vi "Take_it.vi"(8 "error in (no error) 2":errorcluster, 10 "Combo Box":string(combo), 11 "Camera Image":T1) -> (0 "error out":errorcluster, 2 "Done":bool)   [LabVIEW 2019]
uses:
  <vilib>/vision/Image Controls.llb/IMAQ Image.ctl
  Mashina_podyehala.vi
  Camera_angle.vi
  Arm_stage_var.vi
  Timer.vi
  <vilib>/vision/NI_Vision_Development_Module.lvlib
  Simulated Robot/Simulation SubVIs/Simulation SubVIs.lvlib
panel:
  out "New Image":T1
  out "Stage":i32
  out "Threshold":T1(plugin-control)
  out "Raw Image":T1(plugin-control)
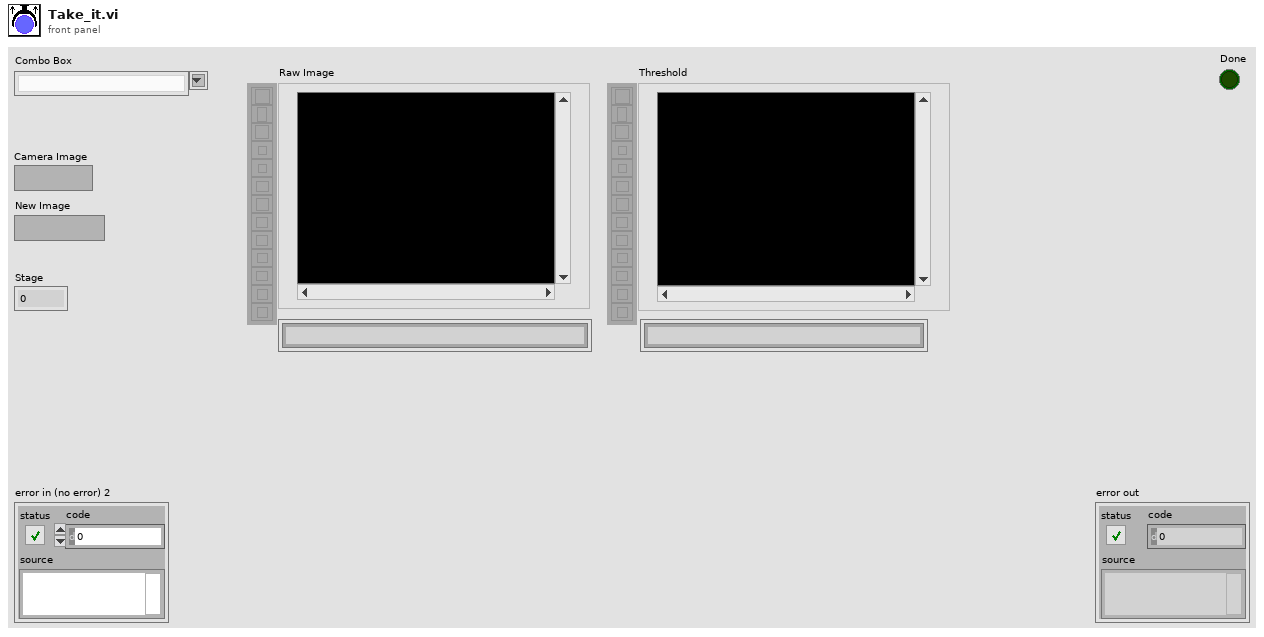
[diagram p1: front panel]
types:
  T1 = typedef "IMAQ Image.ctl" = refnum<image>
  T2 = typedef "Image Type" = u32
  T3 = typedef "Particle Parameters" = i32
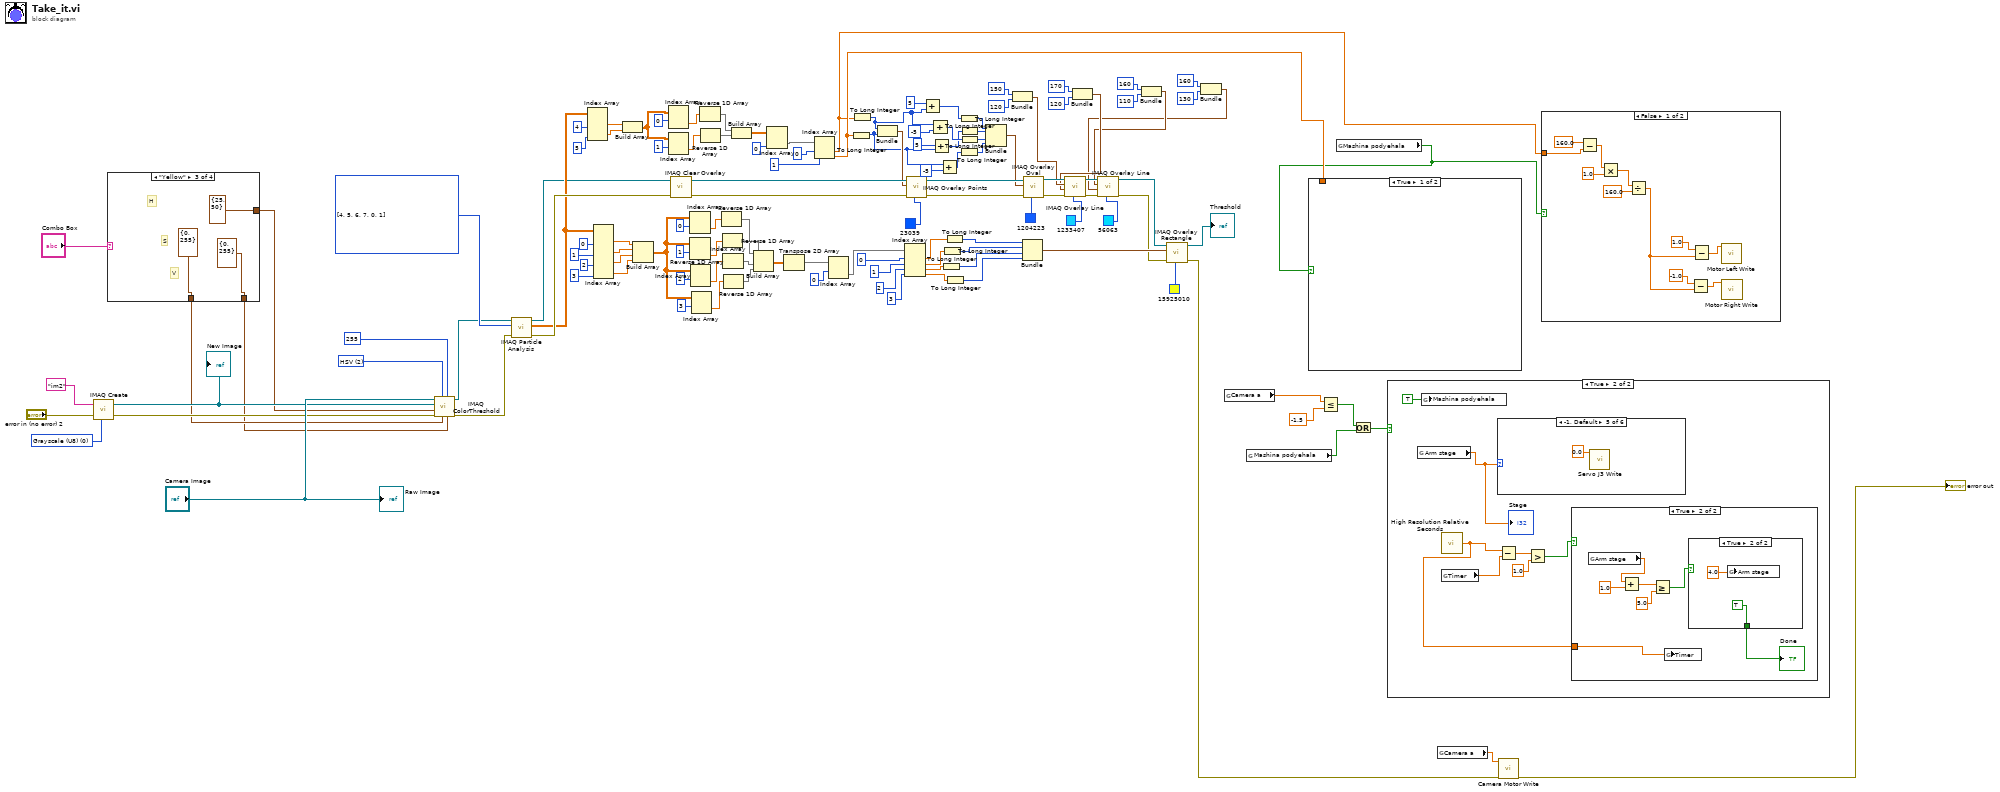
[diagram p0: block diagram]
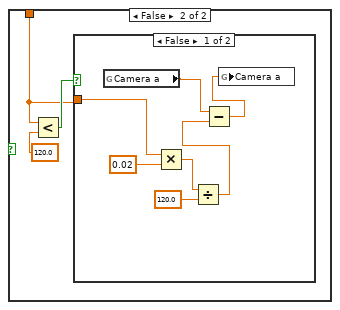
[diagram p2: hidden frame]
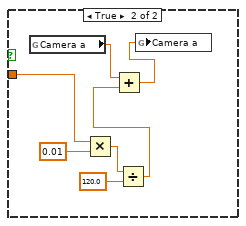
[diagram p3: hidden frame]
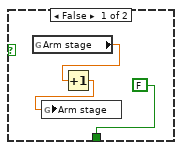
[diagram p6: hidden frame]
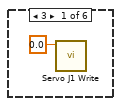
[diagram p7: hidden frame]
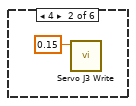
[diagram p8: hidden frame]
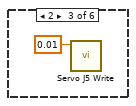
[diagram p9: hidden frame]
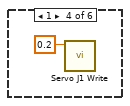
[diagram p10: hidden frame]
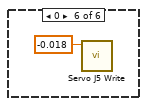
[diagram p11: hidden frame]
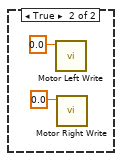
[diagram p12: hidden frame]
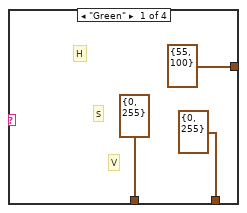
[diagram p13: hidden frame]
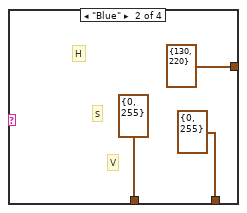
[diagram p14: hidden frame]
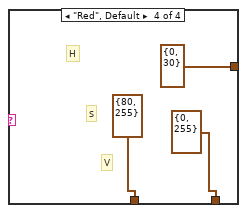
[diagram p15: hidden frame]
diagram:
  w13 = T2 0 items=["Grayscale (U8)", "Grayscale (I16)", "Grayscale (SGL)", "Complex (CSG)", "RGB (U32)", "HSL (U32)", "RGB (U64)", "Grayscale (U16)"] ("Image Type")
  w126 = u16 2 items=["RGB", "HSL", "HSV", "HSI"] ("Color Mode")
  w124 = T3[] [4, 5, 6, 7, 0, 1] items=["Center of Mass X", "Center of Mass Y", "First Pixel X", "First Pixel Y", "Bounding Rect Left", "Bounding Rect Top", "Bounding Rect Right", "Bounding Rect Bottom", "Max Feret Diameter Start X", "Max Feret Diameter Start Y", "Max Feret Diameter End X", "Max Feret Diameter End Y", "Max Horiz. Segment Length Left", "Max Horiz. Segment Length Right", "Max Horiz. Segment Length Row", "-", "Bounding Rect Width", "Bounding Rect Height", "Bounding Rect Diagonal", "Perimeter", "Convex Hull Perimeter", "Holes' Perimeter", "Max Feret Diameter", "Equivalent Ellipse Major Axis", "Equivalent Ellipse Minor Axis", "Equivalent Ellipse Minor Axis (Feret)", "Equivalent Rect Long Side", "Equivalent Rect Short Side", "Equivalent Rect Diagonal", "Equivalent Rect Short Side (Feret)", "Average Horiz. Segment Length", "Average Vert. Segment Length", "Hydraulic Radius", "Waddel Disk Diameter", "-", "Area", "Holes' Area", "Particle & Holes' Area", "Convex Hull Area", "Image Area", "-", "Number of Holes", "Number of Horiz. Segments", "Number of Vert. Segments", "-", "Orientation", "Max Feret Diameter Orientation", "-", "% Area/Image Area", "% Area/(Particle & Holes' Area)", "Ratio of Equivalent Ellipse Axes", "Ratio of Equivalent Rect Sides", "-", "Elongation Factor", "Compactness Factor", "Heywood Circularity Factor", "Type Factor", "-", "Sum X", "Sum Y", "Sum XX", "Sum XY", "Sum YY", "Sum XXX", "Sum XXY", "Sum XYY", "Sum YYY", "-", "Moment of Inertia XX", "Moment of Inertia XY", "Moment of Inertia YY", "Moment of Inertia XXX", "Moment of Inertia XXY", "Moment of Inertia XYY", "Moment of Inertia YYY", "Norm. Moment of Inertia XX", "Norm. Moment of Inertia XY", "Norm. Moment of Inertia YY", "Norm. Moment of Inertia XXX", "Norm. Moment of Inertia XXY", "Norm. Moment of Inertia XYY", "Norm. Moment of Inertia YYY", "Hu Moment 1", "Hu Moment 2", "Hu Moment 3", "Hu Moment 4", "Hu Moment 5", "Hu Moment 6", "Hu Moment 7"] ("Pixel Measurements")
  n1 = call "IMAQ Create"("Image Name"="im2", "Image Type"=w13, "error in (no error)"="error in (no error) 2") -> ("New Image"=w12:T1, "error out"=w9:errorcluster)  [unwired: 2 in]
  "New Image" <- w12
  n2 = case shown="\"Yellow\"" "Combo Box" {
    tunnel: [cluster{"Lower value":i32, "Upper value":i32} {"Lower value"=55, "Upper value"=100} ("Red or Hue Range") cluster{"Lower value":i32, "Upper value":i32} {"Lower value"=130, "Upper value"=220} ("Red or Hue Range") cluster{"Lower value":i32, "Upper value":i32} {"Lower value"=25, "Upper value"=50} ("Red or Hue Range") cluster{"Lower value":i32, "Upper value":i32} {"Lower value"=0, "Upper value"=30} ("Red or Hue Range")] -> w6
    tunnel: [cluster{"Lower value":i32, "Upper value":i32} {"Lower value"=0, "Upper value"=255} ("Green or Sat Range") cluster{"Lower value":i32, "Upper value":i32} {"Lower value"=0, "Upper value"=255} ("Green or Sat Range") cluster{"Lower value":i32, "Upper value":i32} {"Lower value"=0, "Upper value"=255} ("Green or Sat Range") cluster{"Lower value":i32, "Upper value":i32} {"Lower value"=80, "Upper value"=255} ("Green or Sat Range")] -> w5
    tunnel: [cluster{"Lower value":i32, "Upper value":i32} {"Lower value"=0, "Upper value"=255} ("Blue or Luma or Val or Inten Range") cluster{"Lower value":i32, "Upper value":i32} {"Lower value"=0, "Upper value"=255} ("Blue or Luma or Val or Inten Range") cluster{"Lower value":i32, "Upper value":i32} {"Lower value"=0, "Upper value"=255} ("Blue or Luma or Val or Inten Range") cluster{"Lower value":i32, "Upper value":i32} {"Lower value"=0, "Upper value"=255} ("Blue or Luma or Val or Inten Range")] -> w4
    frame "Green" {
      # "V"
      # "S"
      # "H"
    }
    frame "Blue" {
      # "V"
      # "S"
      # "H"
    }
    frame "Yellow" {
      # "V"
      # "S"
      # "H"
    }
    frame "Red", Default {
      # "V"
      # "S"
      # "H"
    }
  }
  n3 = call "IMAQ ColorThreshold"("Blue or Luma or Val or Inten Range"=w4, "Replace Value"=255, "Green or Sat Range"=w5, "Color Mode"=w126, "error in (no error)"=w9, "Red or Hue Range"=w6, "Image Dst"=w12, "Image Src"="Camera Image") -> ("error out"=w19:errorcluster, "Image Dst Out"=w8:T1)  [unwired: 2 in]
  n4 = call "IMAQ Particle Analysis"("error in (no error)"=w19, "Pixel Measurements"=w124, "Image"=w8) -> ("error out"=w25:errorcluster, "Particle Measurements (Pixels)"=w24:dbl[][], "Image Out (duplicate)"=w7:T1)  [unwired: 3 in, 3 out]
  n5 = Index Array(array=w24, index (col) #1=4 ("disabled index (col)"), index (col) #2=5 ("index (col)")) -> (element #1=w74:dbl[], element #2=w73:dbl[])  [unwired: 2 in]
  n6 = Index Array(array=w24, index (col) #1=0 ("disabled index (col)"), index (col) #2=1 ("index (col)"), index (col) #3=2 ("index (col)"), index (col) #4=3 ("index (col)")) -> (element #1=w119:dbl[], element #2=w118:dbl[], element #3=w117:dbl[], element #4=w116:dbl[])  [unwired: 4 in]
  n7 = Build Array(w74, w73) -> (w70:dbl[][])
  n8 = Build Array(w119, w118, w117, w116) -> (w107:dbl[][])
  n9 = Index Array(array=w70, index (row)=0) -> (element=w69:dbl[])  [unwired: 1 in]
  n10 = Index Array(array=w70, index (row)=1) -> (element=w68:dbl[])  [unwired: 1 in]
  n11 = call "IMAQ Clear Overlay"("error in (no error)"=w25, "Image"=w7) -> ("error out"=w63:errorcluster, "Image Out"=w80:T1)  [unwired: 8 in]
  n12 = Index Array(array=w107, index (row)=0) -> (element=w115:dbl[])  [unwired: 1 in]
  n13 = Index Array(array=w107, index (row)=1) -> (element=w114:dbl[])  [unwired: 1 in]
  n14 = Index Array(array=w107, index (row)=2) -> (element=w113:dbl[])  [unwired: 1 in]
  n15 = Index Array(array=w107, index (row)=3) -> (element=w108:dbl[])  [unwired: 1 in]
  n16 = Reverse 1D Array(array=w69) -> (reversed array=w67:dbl[])
  n17 = Reverse 1D Array(array=w68) -> (reversed array=w66:dbl[])
  n18 = Reverse 1D Array(array=w115) -> (reversed array=w111:dbl[])
  n19 = Reverse 1D Array(array=w114) -> (reversed array=w112:dbl[])
  n20 = Reverse 1D Array(array=w113) -> (reversed array=w110:dbl[])
  n21 = Reverse 1D Array(array=w108) -> (reversed array=w109:dbl[])
  n22 = Build Array(w67, w66) -> (w65:dbl[][])
  n23 = Build Array(w111, w112, w110, w109) -> (w102:dbl[][])
  n24 = Index Array(array=w65, index (col)=0 ("index (row)")) -> (element=w79:dbl[])  [unwired: 1 in]
  n25 = Transpose 2D Array(2D array=w102) -> (transposed array=w90:dbl[][])
  n26 = Index Array(array=w79, index #1=0 ("index"), index #2=1 ("index")) -> (element #1=w21:dbl, element #2=w22:dbl)
  n27 = Index Array(array=w90, index (row)=0) -> (element=w89:dbl[])  [unwired: 1 in]
  n28 = To Long Integer(number=w22) -> (32bit integer=w49:i32)
  n29 = To Long Integer(number=w21) -> (32bit integer=w52:i32)
  n30 = Bundle(w52, w49) -> (w75:cluster{i32, i32})  [unwired: 1 in]
  n31 = Index Array(array=w89, index #1=0 ("index"), index #2=1 ("index"), index #3=2 ("index"), index #4=3 ("index")) -> (element #1=w88:dbl, element #2=w87:dbl, element #3=w86:dbl, element #4=w85:dbl)
  n32 = call "IMAQ Overlay Points"("Color"=u32 23039, "error in (no error)"=w63, "Point"=w75, "Image"=w80) -> ("error out"=w62:errorcluster, "Image Out"=w64:T1)  [unwired: 6 in]
  n33 = Add(x=5, y=w52) -> (x+y=w54:i32)
  n34 = Add(x=w52, y=-5) -> (x+y=w53:i32)
  n35 = Add(x=5, y=w49) -> (x+y=w46:i32)
  n36 = Add(x=w49, y=-5) -> (x+y=w47:i32)
  n37 = To Long Integer(number=w86) -> (32bit integer=w93:i32)
  n38 = To Long Integer(number=w87) -> (32bit integer=w94:i32)
  n39 = To Long Integer(number=w88) -> (32bit integer=w95:i32)
  n40 = To Long Integer(number=w85) -> (32bit integer=w92:i32)
  n41 = To Long Integer(number=w54) -> (32bit integer=w56:i32)
  n42 = To Long Integer(number=w47) -> (32bit integer=w57:i32)
  n43 = To Long Integer(number=w46) -> (32bit integer=w59:i32)
  n44 = To Long Integer(number=w53) -> (32bit integer=w58:i32)
  n45 = Bundle(w56, w59, w58, w57) -> (w60:cluster{i32, i32, i32, i32})  [unwired: 1 in]
  n46 = Bundle(150, 120) -> (w35:cluster{i32, i32})  [unwired: 1 in]
  n47 = Bundle(w95, w94, w93, w92) -> (w96:cluster{i32, i32, i32, i32})  [unwired: 1 in]
  n48 = call "IMAQ Overlay Oval"("Color"=u32 1204223, "error in (no error)"=w62, "Bounding Rectangle"=w60, "Image"=w64) -> ("error out"=w44:errorcluster, "Image Out"=w45:T1)  [unwired: 6 in]
  n49 = Bundle(170, 120) -> (w32:cluster{i32, i32})  [unwired: 1 in]
  n50 = call "IMAQ Overlay Line"("Color"=u32 1233407, "error in (no error)"=w44, "End Point"=w32, "Start Point"=w35, "Image"=w45) -> ("error out"=w42:errorcluster, "Image Out"=w43:T1)  [unwired: 5 in]
  n51 = Bundle(160, 110) -> (w27:cluster{i32, i32})  [unwired: 1 in]
  n52 = Bundle(160, 130) -> (w26:cluster{i32, i32})  [unwired: 1 in]
  n53 = call "IMAQ Overlay Line"("Color"=u32 56063, "error in (no error)"=w42, "End Point"=w26, "Start Point"=w27, "Image"=w43) -> ("error out"=w41:errorcluster, "Image Out"=w40:T1)  [unwired: 5 in]
  n54 = call "IMAQ Overlay Rectangle"("Color"=u32 15925010, "error in (no error)"=w41, "Rectangle"=w96, "Image"=w40) -> ("error out"=w20:errorcluster, "Image Out"=→"Threshold":T1)  [unwired: 6 in]
  n55 = global read "Camera_angle.vi" "Camera a"() -> (w17:dbl)
  n56 = global read "Mashina_podyehala.vi" "Mashina podyehala"() -> (w3:bool)
  n57 = Less Or Equal?(x=w17, y=-1.5) -> (x <= y?=w1:bool)
  n58 = global read "Mashina_podyehala.vi" "Mashina podyehala"() -> (w18:bool)
  n59 = case shown="True" w18 {
    tunnel: w22 -> [_ w140]
    frame True {
    }
    frame False {
      n60 = Less?(x=w140, y=120.0) -> (x < y?=w141:bool)
      n61 = case shown="False" w141 {
        tunnel: w140 -> [w148 w152]
        frame False {
          n62 = global read "Camera_angle.vi" "Camera a"() -> (w143:dbl)
          n63 = Multiply(x=w148, y=0.02) -> (x*y=w146:dbl)
          n64 = Divide(x=w146, y=120.0) -> (x/y=w145:dbl)
          n65 = Subtract(x=w143, y=w145) -> (x-y=w144:dbl)
          n66 = global write "Camera_angle.vi" "Camera a"(w144) -> ()
        }
        frame True {
          n67 = global read "Camera_angle.vi" "Camera a"() -> (w150:dbl)
          n68 = Multiply(x=w152, y=0.01) -> (x*y=w154:dbl)
          n69 = Divide(x=w154, y=120.0) -> (x/y=w153:dbl)
          n70 = Add(x=w150, y=w153) -> (x+y=w151:dbl)
          n71 = global write "Camera_angle.vi" "Camera a"(w151) -> ()
        }
      }
    }
  }
  n72 = Or(x=w1, y=w3) -> (x .or. y?=w2:bool)
  n73 = case shown="True" w2 {
    frame False {
    }
    frame True {
      n74 = global read "Arm_stage_var.vi" "Arm stage"() -> (w157:dbl)
      "Stage" <- w157
      n75 = global write "Mashina_podyehala.vi" "Mashina podyehala"(TRUE ("Boolean")) -> ()
      n76 = call <vilib>:"High Resolution Relative Seconds.vi"() -> ("relative seconds"=w160:dbl)
      n77 = global read "Timer.vi" "Timer"() -> (w158:dbl)
      n78 = case shown="-1, Default" w157 {
        frame 3 {
          n79 = call "Servo J1 Write.vi"("J1 Position (m)"=0.0) -> ()  [unwired: 10 in, 1 out]
        }
        frame 4 {
          n80 = call "Servo J3 Write.vi"("J3 Position (m)"=0.15) -> ()  [unwired: 10 in, 1 out]
        }
        frame 2 {
          n81 = call "Servo J5 Write.vi"("J5 Position (m)"=0.01) -> ()  [unwired: 10 in, 1 out]
        }
        frame 1 {
          n82 = call "Servo J1 Write.vi"("J1 Position (m)"=0.2) -> ()  [unwired: 10 in, 1 out]
        }
        frame -1, Default {
          n83 = call "Servo J3 Write.vi"("J3 Position (m)"=0.0) -> ()  [unwired: 10 in, 1 out]
        }
        frame 0 {
          n84 = call "Servo J5 Write.vi"("J5 Position (m)"=-0.018) -> ()  [unwired: 10 in, 1 out]
        }
      }
      n85 = Subtract(x=w160, y=w158) -> (x-y=w163:dbl)
      n86 = Greater?(x=w163, y=1.0) -> (0:w161:bool)
      n87 = case shown="True" w161 {
        tunnel: w160 -> [_ w165]
        frame False {
        }
        frame True {
          n88 = global read "Arm_stage_var.vi" "Arm stage"() -> (w166:dbl)
          n89 = Add(x=w166, y=1.0) -> (x+y=w169:dbl)
          n90 = Greater Or Equal?(x=w169, y=5.0) -> (x >= y?=w168:bool)
          n91 = global write "Timer.vi" "Timer"(w165) -> ()
          n92 = case shown="True" w168 {
            tunnel: [FALSE ("Done") TRUE ("Done")] -> w164
            frame False {
              n93 = global read "Arm_stage_var.vi" "Arm stage"() -> (w173:dbl)
              n94 = Increment(x=w173) -> (x+1=w172:dbl)
              n95 = global write "Arm_stage_var.vi" "Arm stage"(w172) -> ()
            }
            frame True {
              n96 = global write "Arm_stage_var.vi" "Arm stage"(4.0 ("Numeric")) -> ()
            }
          }
          "Done" <- w164
        }
      }
    }
  }
  n97 = global read "Camera_angle.vi" "Camera a"() -> (w16:dbl)
  n98 = call "Camera Motor Write.vi"("error in (no error)"=w20, "Camera Position (rad)"=w16) -> ("error out"=→"error out":errorcluster)  [unwired: 9 in]
  n99 = case shown="False" w18 {
    tunnel: w21 -> [w183 _]
    frame False {
      n100 = Subtract(x=160.0, y=w183) -> (x-y=w182:dbl)
      n101 = Multiply(x=w182, y=1.0) -> (x*y=w191:dbl)
      n102 = Divide(x=w191, y=160.0) -> (x/y=w192:dbl)
      n103 = Subtract(x=-1.0, y=w192) -> (x-y=w190:dbl)
      n104 = Subtract(x=1.0, y=w192) -> (x-y=w189:dbl)
      n105 = call "Motor Left Write.vi"("left motor ccw velocity (rad/s)"=w189) -> ()  [unwired: 10 in, 1 out]
      n106 = call "Motor Right Write.vi"("right motor ccw velocity (rad/s)"=w190) -> ()  [unwired: 10 in, 1 out]
    }
    frame True {
      n107 = call "Motor Left Write.vi"("left motor ccw velocity (rad/s)"=0.0) -> ()  [unwired: 10 in, 1 out]
      n108 = call "Motor Right Write.vi"("right motor ccw velocity (rad/s)"=0.0) -> ()  [unwired: 10 in, 1 out]
    }
  }
  "Raw Image" <- "Camera Image"
